vi "Configure Device.vi"(8 "error in":errorcluster, 11 "Alicat Device In":refnum<class "Alicat Device.lvclass">) -> (0 "error out":errorcluster, 3 "Alicat Device Out":refnum<class "Alicat Device.lvclass">, 4 "SP":dbl, 5 "Settable?":bool)   [LabVIEW 2018, in "Alicat Lib.lvlib" / "Alicat Device.lvclass"]
doc: "Configure the serial port for communication with the Alicat devices. We will create new Alicat objects based upon an input array of addresses. If an address is no good, then we will delete the session reference and move onto the next address. We determine if the session is good by sending a request for data to the device until the device \"wakes up\" and responds properly. If the device does not repsond properly, then set the boolean property <b>Active</b> to alert potential callers that this instantiation is non-communicative.\n\nAlthough the caller can configure the port with the desired serial and message settings, the default settings should be sufficient for most applications."
uses:
  Alicat Device.lvclass
  reusable/Session APIs/Serial/Serial Session.lvclass
  reusable/Session APIs/File Access/Config Data/Config Data.lvclass
  <vilib>/Utility/config.llb/NI_LVConfig.lvlib
  <vilib>/Utility/config.llb/Read Key (String).vi
  <vilib>/Utility/config.llb/Read Key (Double).vi
  Configurable Device/Configurable Device.lvclass
  <userlib>/_Session Fwk/Session - Root.lvclass
  <vilib>/ErrorRing/Error Ring.xnode
  reusable/Session APIs/Session Log/System Log.lvclass
  Data/Alicat Data.lvclass
  C:/Users/Labview/Documents/exscalabar_server/Devices/Configurable Device/Configurable Device.lvclass
  C:/Program Files (x86)/National Instruments/LabVIEW 2018/user.lib/_Session Fwk/Session - Root.lvclass
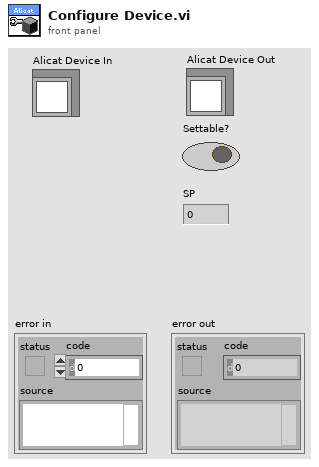
[diagram p1: front panel]
types:
  T1 = typedef "Serial Session.lvclass/Session Handle.ctl" = refnum<data-value>
  T2 = typedef "Config Data.lvclass/Config Session.ctl" = refnum<data-value>
  T3 = typedef "Session - Root.lvclass/Session Handle.ctl" = refnum<data-value>
  T4 = typedef "NI_LVConfig.lvlib/Config Data RefNum.ctl" = refnum<k1>
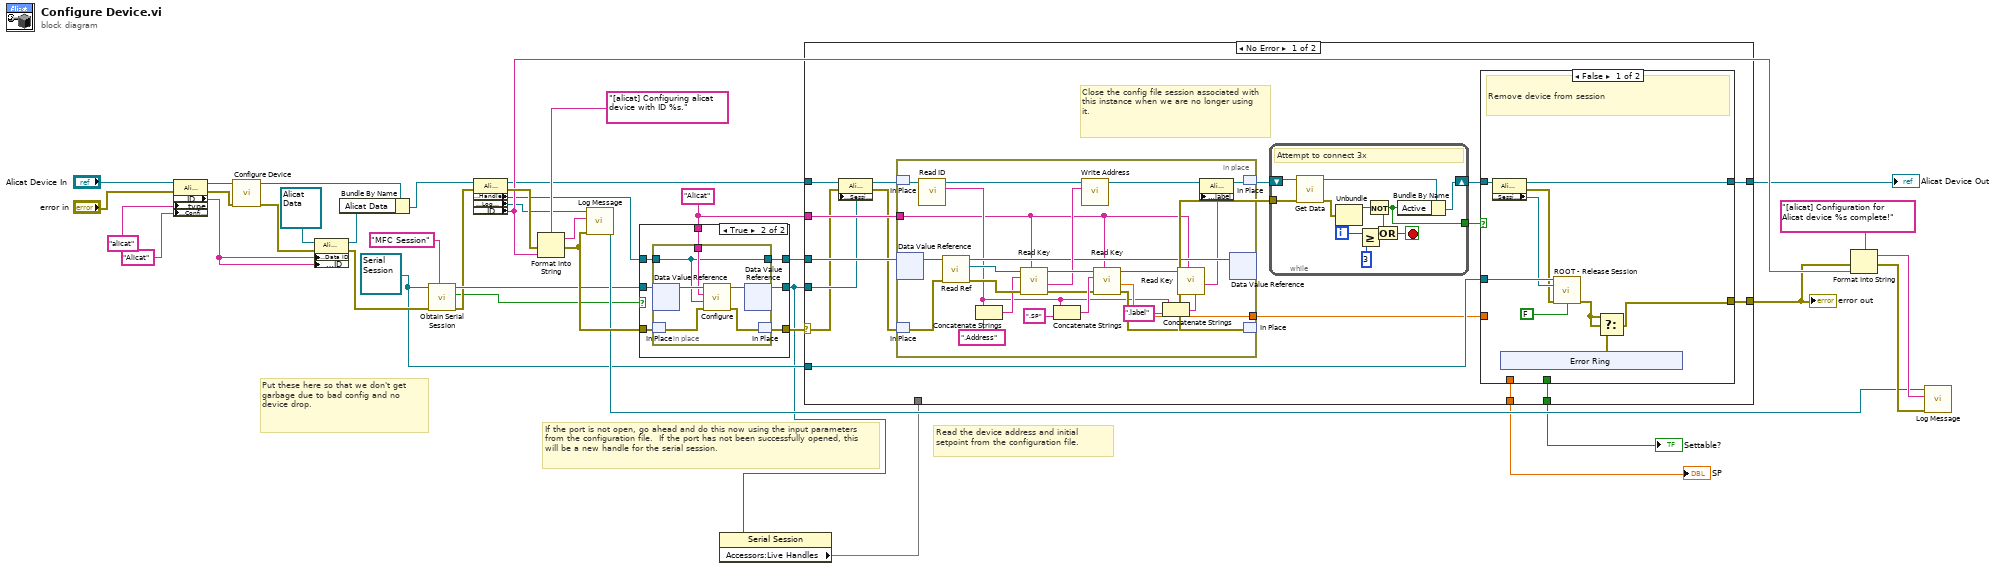
[diagram p0: block diagram]
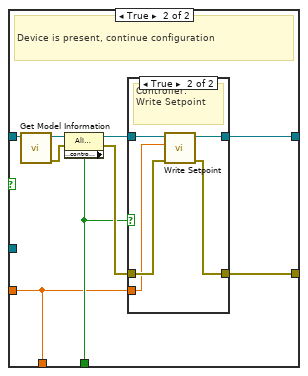
[diagram p2: hidden frame]
diagram:
  w21 = refnum<class "Serial Session.lvclass"> refnum ("Serial Session in")
  w19 = "Alicat" ("section")
  # "Put these here so that we don't get garbage due to bad config and no device drop."
  # "If the port is not open, go ahead and do this now using the input parameters from the configuration file.  If the port has not been successfully opened, this will be a new handle for the serial session."
  # "Read the device address and initial setpoint from the configuration file."
  n1 = property class="Alicat Device"(reference="Alicat Device In", error in="error in", "Accessors:type"="alicat" ("type"), "Accessors:Config Section"="Alicat" ("section")) -> (reference out=w6:refnum<class "Alicat Device.lvclass">, error out=w5:errorcluster, "Accessors:ID"=w33:string)
  n2 = call-parent "Configure Device.vi"("error in"=w5, "Device in"=w6) -> ("error out"=w4:errorcluster, "Device out"=w3:refnum<class "Alicat Device.lvclass">)  [unwired: 6 in, 2 out]
  n3 = property class="Alicat Data"(reference=refnum<class "Alicat Data.lvclass"> refnum ("Alicat Lib.lvlib:Alicat Data"), error in=w4, "Accessors:Data ID"=w33, "Accessors:ID"=w33) -> (reference out=w35:refnum<class "Alicat Data.lvclass">, error out=w36:errorcluster)
  n4 = Bundle By Name(cluster=w3, "Alicat Data"=w35) -> (w34:refnum<class "Alicat Device.lvclass">)
  n5 = call "Obtain Serial Session.vi"("Session Name ()"="MFC Session", "error in"=w36, "Serial Session in"=w21) -> ("error out"=w17:errorcluster, "created new?"=w14:bool, "hSerial"=w20:T1)  [unwired: 6 in]
  n6 = property class="Alicat Device"(reference=w34, error in=w17) -> (reference out=w22:refnum<class "Alicat Device.lvclass">, error out=w37:errorcluster, "Accessors:Handle"=w16:T2, "Accessors:Log Session"=w24:T3, "Accessors:ID"=w31:string)
  n7 = Format Into String(format string="[alicat] Configuring alicat device with ID %s.", error in=w37, w31) -> (resulting string=w26:string, error out=w38:errorcluster)  [unwired: 1 in]
  n8 = call "Log Message.vi"("error in"=w38, "MSG In"=w26, "session in"=w24) -> ("session out"=w27:T3)  [unwired: 7 in, 1 out]
  n9 = case shown="True" w14 {
    tunnel: w20 -> [w42 w49]
    tunnel: w38 -> [w41 w45]
    tunnel: [w42 w48] -> w2
    tunnel: [w41 w47] -> w23
    tunnel: w16 -> [w40 w46]
    tunnel: [w40 w44] -> w18
    tunnel: w19 -> [_ w43]
    frame False {
    }
    frame True {
      n10 = in-place {
        in-place-border: w46 -> [w50]
        in-place-border: w43 -> [w51]
        in-place-border: [w50] -> w44
        n11 = in-place-dvr #1(w49) -> (w55:refnum<class "Serial Session.lvclass">)  [unwired: 1 out]
        n12 = in-place-match #2(w45) -> (w54:errorcluster)
        n13 = call "Configure.vi"("error in"=w54, "Config Handle"=w50, "section"=w51, "Serial Session in"=w55) -> ("error out"=w53:errorcluster, "Serial Session out"=w52:refnum<class "Serial Session.lvclass">)  [unwired: 6 in]
        n14 = in-place-dvr #1(w52) -> (w48:T1)  [unwired: 1 out]
        n15 = in-place-match #2(w53) -> (w47:errorcluster)
      }
    }
  }
  n16 = property class="Serial Session"(reference=w2) -> ("Accessors:Live Handles"=w1)  [unwired: 1 in, 2 out]
  n17 = case shown="No Error" w23 {
    selector: w23 -> [w60 w134]
    tunnel: w18 -> [w72 _]
    tunnel: w19 -> [w71 _]
    tunnel: w21 -> [w70 _]
    tunnel: [w68 w134] -> w9
    tunnel: [w65 w135] -> w10
    tunnel: w22 -> [w64 w135]
    tunnel: w2 -> [w62 _]
    tunnel: [w57 _] -> w8
    tunnel: [w56 _] -> w7
    tunnel: w1 -> [_ _]
    frame No Error {
      # "Close the config file session associated with this instance when we are no longer using it."
      n18 = property class="Alicat Device"(reference=w64, error in=w60, "Accessors:Session Handle"=w62) -> (reference out=w63:refnum<class "Alicat Device.lvclass">, error out=w61:errorcluster)
      n19 = in-place {
        in-place-border: w71 -> [w110]
        in-place-border: [w122] -> w66
        n20 = in-place-match #3(w63) -> (w120:refnum<class "Alicat Device.lvclass">)
        n21 = in-place-dvr #4(w72) -> (w133:refnum<class "Config Data.lvclass">)  [unwired: 1 out]
        n22 = in-place-match #5(w61) -> (w132:errorcluster)
        n23 = call "Read ID.vi"("Configurable Device in"=w120) -> ("ID"=w113:string, "Configurable Device out"=w119:refnum<class "Alicat Device.lvclass">)  [unwired: 8 in, 1 out]
        n24 = call "Read Ref.vi"("error in"=w132, "Config Data in"=w133) -> ("error out"=w130:errorcluster, "config data"=w131:T4, "Config Data out"=w121:refnum<class "Config Data.lvclass">)  [unwired: 7 in]
        n25 = Concatenate Strings(w113, ".Address" ("string")) -> (w128:string)
        n26 = call-poly <vilib>:"Read Key.vi"("section"=w110, "error in (no error)"=w130, "key"=w128, "refnum"=w131) -> ("error out"=w124:errorcluster, "value"=w123:string, "refnum out"=w127:T4)  [unwired: 4 in, 1 out]
        n27 = Concatenate Strings(w113, ".SP" ("string")) -> (w125:string)
        n28 = call "Write Address.vi"("Address"=w123, "Alicat Device in"=w119) -> ("Alicat Device out"=w117:refnum<class "Alicat Device.lvclass">)  [unwired: 8 in, 1 out]
        n29 = call-poly <vilib>:"Read Key.vi"("section"=w110, "error in (no error)"=w124, "key"=w125, "refnum"=w127) -> ("error out"=w118:errorcluster, "value"=w122:dbl, "refnum out"=w112:T4)  [unwired: 4 in, 1 out]
        n30 = Concatenate Strings(w113, ".label" ("string")) -> (w114:string)
        n31 = call-poly <vilib>:"Read Key.vi"("section"=w110, "key"=w114, "refnum"=w112) -> ("value"=w111:string)  [unwired: 5 in, 3 out]
        n32 = property class="Alicat Device"(reference=w117, "Accessors:label"=w111) -> (reference out=w116:refnum<class "Alicat Device.lvclass">)  [unwired: 1 in, 1 out]
        n33 = in-place-dvr #4(w121) -> ()  [unwired: 2 out]
        n34 = in-place-match #3(w116) -> (w69:refnum<class "Alicat Device.lvclass">)
        n35 = in-place-match #5(w118) -> (w58:errorcluster)
      }
      n36 = while {
        tunnel: w58 -> [w104]
        shift-right: [w102] -> w67
        shift-left: w69 -> [w105]
        tunnel: [w101] -> w59
        i -> [w99]
        stop <- w106 stop-if-true
        # "Attempt to connect 3x"
        n37 = call-dynamic "Get Data.vi"("error in"=w104, "Alicat Device in"=w105) -> ("error out"=w100:errorcluster, "Alicat Device out"=w103:refnum<class "Alicat Device.lvclass">)  [unwired: 7 in, 1 out]
        n38 = Unbundle(w100) -> ("status"=w107:bool)  [unwired: 2 out]
        n39 = Greater Or Equal?(x=w99, y=3) -> (x >= y?=w108:bool)
        n40 = Not(x=w107) -> (.not. x?=w101:bool)
        n41 = Or(x=w101, y=w108) -> (x .or. y?=w106:bool)
        n42 = Bundle By Name(cluster=w103, "Active"=w101) -> (w102:refnum<class "Alicat Device.lvclass">)
      }
      n43 = case shown="False" w59 {
        tunnel: [w73 w90] -> w68
        tunnel: w70 -> [w81 _]
        tunnel: w67 -> [w79 w91]
        tunnel: w66 -> [_ w83]
        tunnel: [w78 w89] -> w65
        tunnel: [_ w84] -> w57
        tunnel: [_ w83] -> w56
        frame False {
          # "Remove device from session"
          n44 = property class="Alicat Device"(reference=w79) -> (reference out=w78:refnum<class "Alicat Device.lvclass">, error out=w76:errorcluster, "Accessors:Session Handle"=w77:T1)  [unwired: 1 in]
          n45 = xnode "Error Ring"() -> ("error out"=w74:errorcluster)
          n46 = call <userlib>:"ROOT - Release Session.vi"("OBJ - Session in"=w81, "Session Handle in"=w77, "error in (no error)"=w76, "force destroy? (F)"=FALSE) -> ("error out"=w75:errorcluster)  [unwired: 10 in, 1 out]
          n47 = Select(t=w75, s=w75, f=w74) -> (s? t:f=w73:errorcluster)
        }
        frame True {
          # "Device is present, continue configuration"
          n48 = call "Get Model Information.vi"("Alicat Device in"=w91) -> ("error out"=w85:errorcluster, "Alicat Device out"=w88:refnum<class "Alicat Device.lvclass">)  [unwired: 7 in, 2 out]
          n49 = property class="Alicat Device"(reference=w88, error in=w85) -> (reference out=w87:refnum<class "Alicat Device.lvclass">, error out=w86:errorcluster, "Accessors:controller_"=w84:bool)
          n50 = case shown="True" w84 {
            tunnel: w86 -> [w92 w97]
            tunnel: w87 -> [w93 w98]
            tunnel: w83 -> [_ w94]
            tunnel: [w92 w96] -> w90
            tunnel: [w93 w95] -> w89
            frame False {
            }
            frame True {
              # "Controller:\nWrite Setpoint"
              n51 = call "Write Setpoint.vi"("error in"=w97, "Setpoint"=w94, "Alicat Device in"=w98) -> ("error out"=w96:errorcluster, "Alicat Device out"=w95:refnum<class "Alicat Device.lvclass">)  [unwired: 6 in, 1 out]
            }
          }
        }
      }
    }
    frame Error {
    }
  }
  "error out" <- w9
  "Alicat Device Out" <- w10
  "Settable?" <- w8
  "SP" <- w7
  n52 = Format Into String(format string="[alicat] Configuration for Alicat device %s complete!", error in=w9, w31) -> (resulting string=w29:string, error out=w30:errorcluster)  [unwired: 1 in]
  n53 = call "Log Message.vi"("error in"=w30, "MSG In"=w29, "session in"=w27) -> ()  [unwired: 7 in, 2 out]
